vi "Read Next.vi"(8 "error in (no error)":errorcluster, 11 "Timeout in":refnum<class "Timeout.lvclass">) -> (0 "error out":errorcluster, 2 "Next":i32, 3 "Timeout out":refnum<class "Timeout.lvclass">)   [LabVIEW 2020, in "Timeout.lvclass"]
uses:
  Timeout.lvclass
  Timeout.lvclass/Timeout.ctl
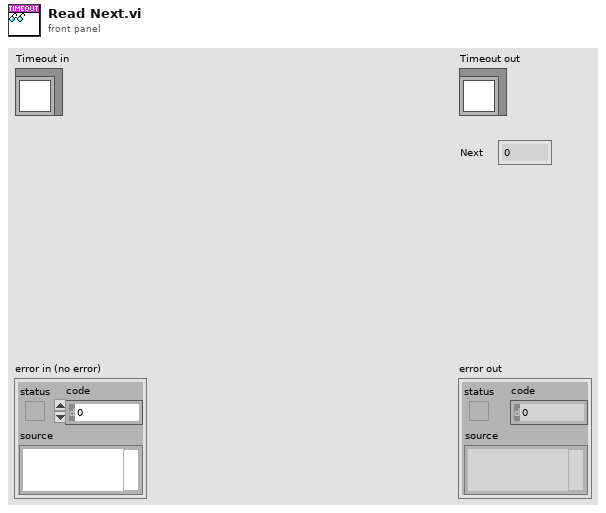
[diagram p1: front panel]
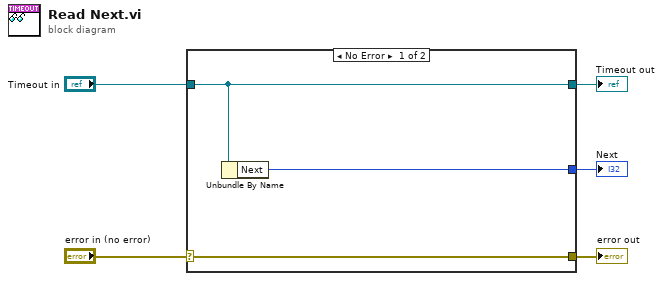
[diagram p0: block diagram]
diagram:
  n1 = case shown="No Error" "error in (no error)" {
    selector: "error in (no error)" -> [w8 w9]
    tunnel: [w8 w9] -> w4
    tunnel: [w7 w10] -> w2
    tunnel: "Timeout in" -> [w7 w10]
    tunnel: [w6 _] -> w1
    frame No Error {
      n2 = Unbundle By Name(w7) -> ("Next"=w6:i32)
    }
    frame Error {
    }
  }
  "error out" <- w4
  "Timeout out" <- w2
  "Next" <- w1
